vi "GPIB_USB_WRITE+DEL READ_VISA IN_OUT(SubVI).vi"(0 "VISA resource IN":refnum<visa-resource-name>, 1 "BYTE COUNT":u32, 2 "GPIB/USB WRITE":string, 3 "DELAY BEFORE READ":u32, 4 "?":bool, 5 "error in (no error)":errorcluster) -> (6 "VISA resource OUT":refnum<visa-resource-name>, 7 "GPIB/USB READ":string, 8 "error out":errorcluster)   [LabVIEW 2011]
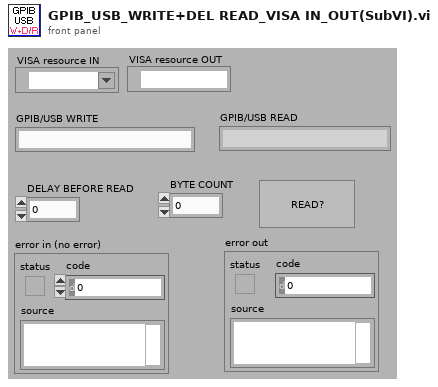
[diagram p1: front panel]
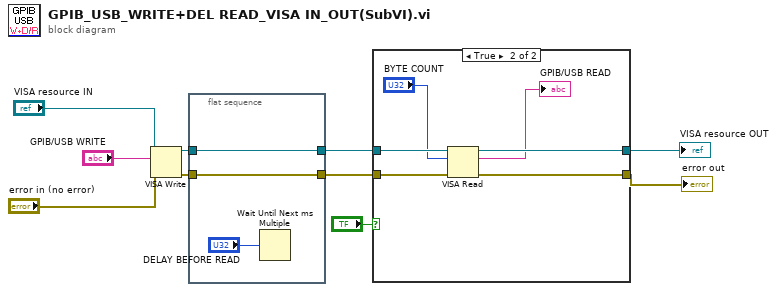
[diagram p0: block diagram]
diagram:
  n1 = VISA Write(VISA resource name="VISA resource IN", write buffer="GPIB/USB WRITE", error in (no error)="error in (no error)") -> (VISA resource name out=w3:refnum<visa-resource-name>, error out=w5:errorcluster)  [unwired: 1 out]
  n2 = flat-sequence {
    tunnel: w3 -> [w13]
    tunnel: [w13] -> w4
    tunnel: w5 -> [w12]
    tunnel: [w12] -> w6
    frame #0 {
      n3 = Wait Until Next ms Multiple(millisecond multiple="DELAY BEFORE READ") -> ()  [unwired: 1 out]
    }
  }
  n4 = case shown="True" "?" {
    tunnel: w4 -> [w15 w21]
    tunnel: w6 -> [w14 w20]
    tunnel: [w15 w19] -> w10
    tunnel: [w14 w18] -> w8
    frame False {
    }
    frame True {
      n5 = VISA Read(VISA resource name=w21, byte count="BYTE COUNT", error in (no error)=w20) -> (VISA resource name out=w19:refnum<visa-resource-name>, read buffer=→"GPIB/USB READ":string, error out=w18:errorcluster)  [unwired: 1 out]
    }
  }
  "error out" <- w8
  "VISA resource OUT" <- w10
